vi "TxChannel - Remove Tx Channels.vi"(8 "error in (no error)":errorcluster, 11 "Node Ptr":T1 format="%.0x") -> (0 "error out":errorcluster)   [LabVIEW 2019, in "UDP-Custom-Device System Explorer.lvlib"]
uses:
  UDP-Custom-Device System Explorer.lvlib
  <vilib>/NI VeriStand/Custom Device API/Custom Device Item Ref.ctl
  Property Accessors/Shared Packet Accessors.lvlib
  <vilib>/NI VeriStand/Custom Device API/Custom Device API.lvlib
  Property Accessors/Tx Channel Section Accessors.lvlib
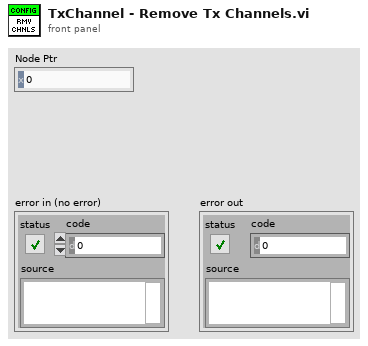
[diagram p1: front panel]
types:
  T1 = typedef "Custom Device API.lvlib/Custom Device Item Ref.ctl" = u64
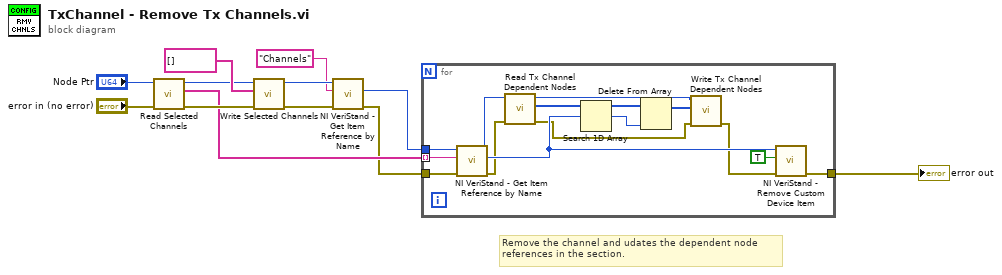
[diagram p0: block diagram]
diagram:
  # "Remove the channel and udates the dependent node\nreferences in the section."
  n1 = call "Read Selected Channels.vi"("error in (no error)"="error in (no error)", "Node Ptr"="Node Ptr") -> ("error out"=w10:errorcluster, "Selected Channel Names"=w8:string[], "Node Ptr out"=w9:T1)  [unwired: 7 in]
  n2 = call "Write Selected Channels.vi"("error in (no error)"=w10, "Selected Channel Names"=string[] [] ("Selected Channel References"), "Node Ptr"=w9) -> ("error out"=w5:errorcluster, "Node Ptr out"=w3:T1)  [unwired: 7 in]
  n3 = call <vilib>:"NI VeriStand - Get Item Reference by Name.vi"("error in (no error)"=w5, "Item Name"="Channels" ("Numeric"), "Parent Ref in"=w3) -> ("error out"=w4:errorcluster, "Item Ref"=w2:T1)  [unwired: 5 in, 2 out]
  n4 = for {
    tunnel: w8 -> [w23] mode=indexing
    tunnel: w4 -> [w22]
    tunnel: [w26] -> w7
    tunnel: w2 -> [w24]
    n5 = call <vilib>:"NI VeriStand - Get Item Reference by Name.vi"("error in (no error)"=w22, "Item Name"=w23, "Parent Ref in"=w24) -> ("error out"=w18:errorcluster, "Item Ref"=w21:T1, "Parent Ref out"=w19:T1)  [unwired: 5 in, 1 out]
    n6 = call "Read Tx Channel Dependent Nodes.vi"("error in (no error)"=w18, "Node Ptr"=w19) -> ("error out"=w14:errorcluster, "Dependent Node Refs"=w17:T1[], "Node Ptr out"=w15:T1)  [unwired: 7 in]
    n7 = Search 1D Array(1D array=w17, element=w21) -> (index of element=w20:i32)  [unwired: 1 in]
    n8 = Delete From Array(array=w17, index=w20) -> (array with subset deleted=w16:T1[])  [unwired: 1 in, 1 out]
    n9 = call "Write Tx Channel Dependent Nodes.vi"("error in (no error)"=w14, "Dependent Node Refs"=w16, "Node Ptr"=w15) -> ("error out"=w13:errorcluster)  [unwired: 7 in, 1 out]
    n10 = call <vilib>:"NI VeriStand - Remove Custom Device Item.vi"("error in (no error)"=w13, "Force Delete (F)"=TRUE, "Item Ref in"=w21) -> ("error out"=w26:errorcluster)  [unwired: 7 in, 1 out]
  }
  "error out" <- w7
